vi "debug_gcode.vi"() -> ()   [LabVIEW 2021]
panel:
  out "subarray":dbl[][](array[numeric])
  out "size(s)":i32[](array[numeric])
  out "element":string
  out "Array":string[](array[string])
  in  "file path (use dialog)":path
  out "array":dbl[][](array[numeric])
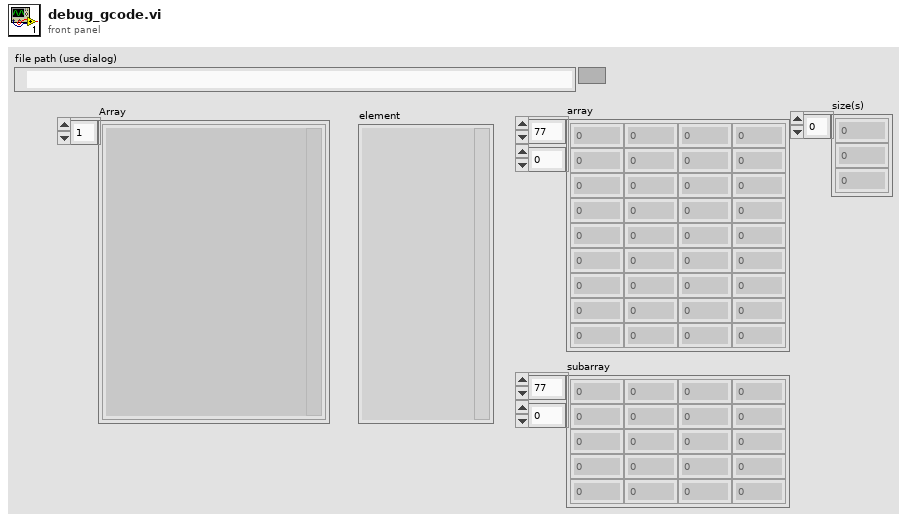
[diagram p1: front panel]
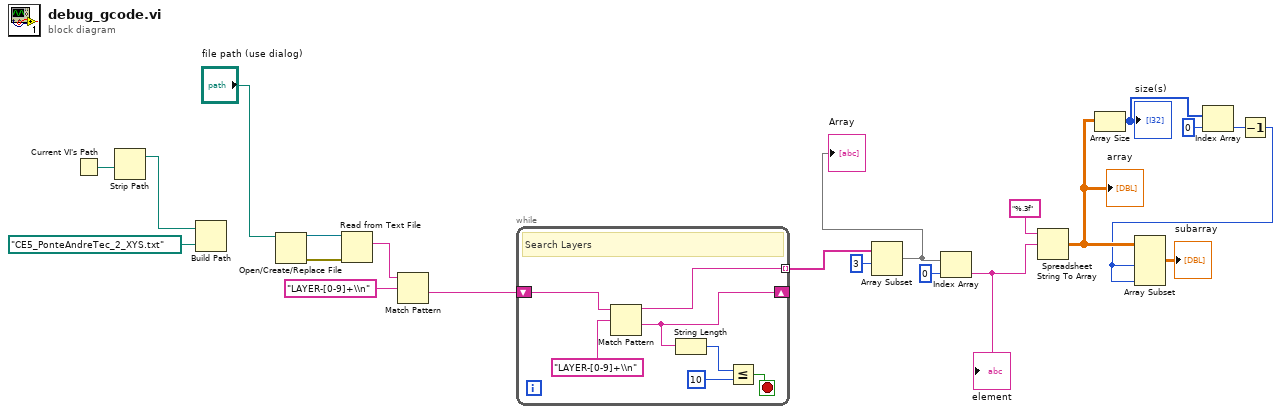
[diagram p0: block diagram]
diagram:
  n1 = Current VI's Path() -> (path=w15:path)
  n2 = Strip Path(path=w15) -> (stripped path=w14:path)  [unwired: 1 out]
  n3 = Build Path(base path=w14, name or relative path=path "CE5_PonteAndreTec_2_XYS.txt" ("file path (use dialog)")) -> ()  [unwired: 1 out]
  n4 = Open/Create/Replace File(file path (use dialog)="file path (use dialog)") -> (refnum out=w20:refnum<file>, error out=w21:errorcluster)  [unwired: 5 in, 1 out]
  n5 = Read from Text File(file (use dialog)=w20, error in=w21) -> (text=w19:string)  [unwired: 2 in, 3 out]
  n6 = Match Pattern(string=w19, regular expression="LAYER-[0-9]+\\n") -> (after substring=w17:string)  [unwired: 1 in, 3 out]
  n7 = while {
    shift-right: [w25] -> _
    shift-left: w17 -> [w27]
    tunnel: [w22] -> w13 mode=indexing
    stop <- w23 stop-if-true
    # "Search Layers"
    n8 = Match Pattern(string=w27, regular expression="LAYER-[0-9]+\\n") -> (before substring=w22:string, after substring=w25:string)  [unwired: 1 in, 2 out]
    n9 = String Length(string=w25) -> (length=w26:i32)
    n10 = Less Or Equal?(x=w26, y=10) -> (x <= y?=w23:bool)
  }
  n11 = Array Subset(array=w13, index=3) -> (w8:string[])  [unwired: 1 in]
  "Array" <- w8
  n12 = Index Array(array=w8, index=0) -> (element=w7:string)
  "element" <- w7
  n13 = Spreadsheet String To Array(format string="%.3f", spreadsheet string=w7) -> (array=w6:dbl[][])  [unwired: 2 in]
  "array" <- w6
  n14 = Array Size(array=w6) -> (size(s)=w4:i32[])
  "size(s)" <- w4
  n15 = Index Array(array=w4, index=0) -> (element=w2:i32)
  n16 = Decrement(x=w2) -> (x-1=w1:i32)
  n17 = Array Subset(array=w6, length (row)=w1, length (col)=w1) -> (→"subarray":dbl[][])  [unwired: 2 in]
